vi "Method.vi"(4 "Abs_Types.lvlib:Numeric.lvclass":refnum<class "Abs_Numeric.lvclass">, 5 "Input A":refnum<class "Abs_Double Float.lvclass">) -> (1 "Result":refnum<class "Abs_Double Float.lvclass">)   [LabVIEW 2021, in "Add_DBL.lvclass"]
uses:
  Add_DBL.lvclass
  Abs_Types/Double Float/Abs_Double Float.lvclass
  Abs_Types/Numeric/Abs_Numeric.lvclass
  C:/TSA/LV_Abstract/Source/Functions/Support/Function/Two Terminal/DBL/AbsFunc_Two Term_DBL.lvclass
  C:/Program Files (x86)/National Instruments/LabVIEW 2021/vi.lib/TSA/Abstract Data Classes/Abs_Types/Double Float/Abs_Double Float.lvclass
  Support/Function/Two Terminal/DBL/AbsFunc_Two Term_DBL.lvclass/AbsFunc_Two Term_DBL.ctl
  Support/Function/Two Terminal/DBL/Properties/Write Numeric A.vi
  Support/Function/Two Terminal/DBL/Properties/Write Numeric B.vi
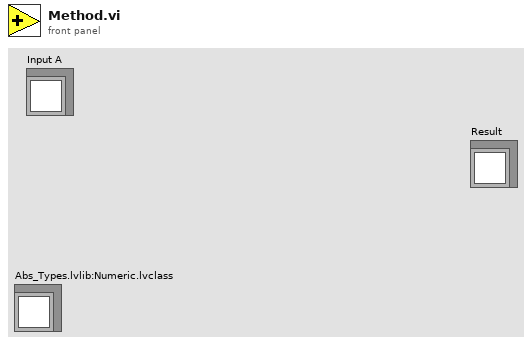
[diagram p1: front panel]
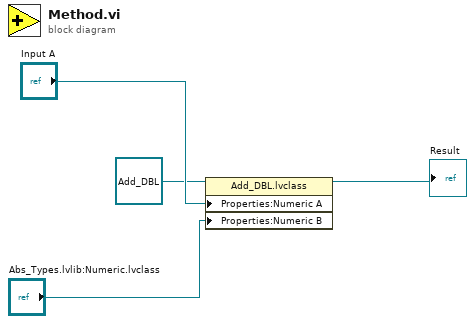
[diagram p0: block diagram]
diagram:
  n1 = property class="Add_DBL.lvclass"(reference=refnum<class "Add_DBL.lvclass"> refnum ("Functions.lvlib:Numeric.lvlib:Add_DBL.lvclass"), "Properties:Numeric A"="Input A", "Properties:Numeric B"="Abs_Types.lvlib:Numeric.lvclass") -> (reference out=→"Result":refnum<class "Add_DBL.lvclass">)  [unwired: 1 in, 1 out]
